vi "Setup Digitizer.vi"(7 "moduleID":i32, 8 "error in (no error)":errorcluster, 9 "Channel M":T1, 10 "DAQ M":T2, 11 "nChannel":i32) -> (0 "error out":errorcluster, 3 "Digitizer ID":i32)   [LabVIEW 2021]
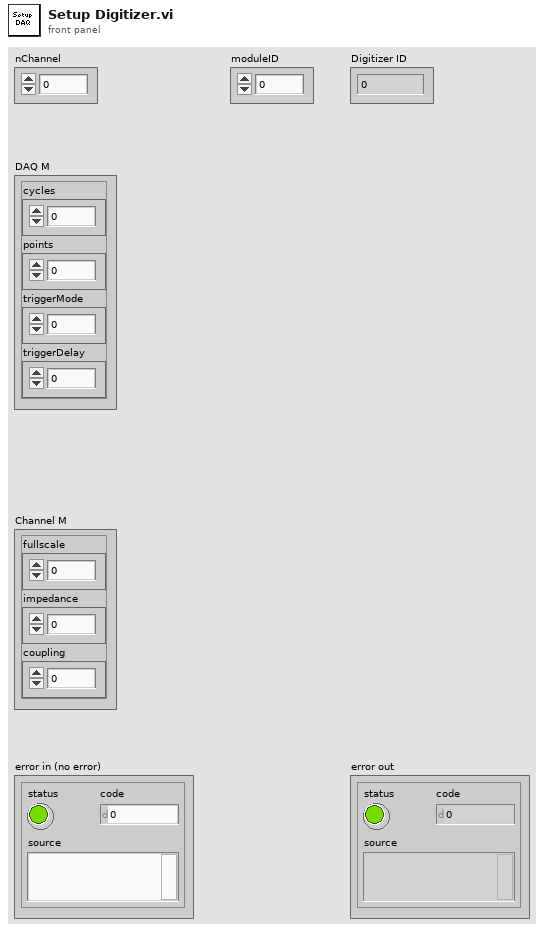
[diagram p1: front panel]
types:
  T1 = cluster{"fullscale":dbl, "impedance":i32, "coupling":i32}
  T2 = cluster{"cycles":i32, "points":i32, "triggerMode":i32, "triggerDelay":i32}
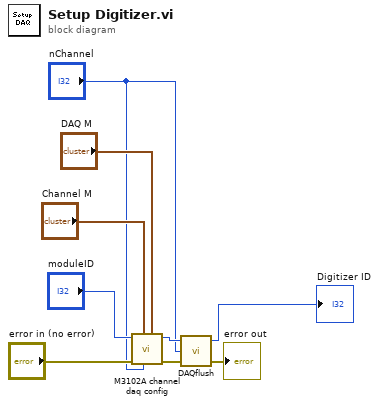
[diagram p0: block diagram]
diagram:
  n1 = call "M3102A channel daq config.vi"("DAQ"="DAQ M", "nChannel"="nChannel", "Channel"="Channel M", "errorIn"="error in (no error)", "moduleID"="moduleID") -> ("errorOut"=w8:errorcluster, "moduleIDout"=w9:i32)  [unwired: 5 in]
  n2 = call <vilib>:"DAQflush.vi"("errorIn"=w8, "nDAQ"="nChannel", "moduleID"=w9) -> ("errorOut"=→"error out":errorcluster, "moduleIDout"=→"Digitizer ID":i32)  [unwired: 1 in]
